vi "DataTransmissionActions.vi"(0 "Action":T2(ring), 1 "Transmission State In":T3(ring), 5 "Port Number In":dbl, 7 "Channel Names In":string[](array[string]), 9 "Time String":string, 11 "error in (no error)":errorcluster, 12 "Total Data In":dbl[](array[numeric]), 13 "Contol\nPoint\nSuffix":T1) -> (3 "Transmission State Out":T3(ring), 4 "Enabled":bool, 6 "Port Number Out":dbl, 10 "Channel Names Out":string[](array[string]), 14 "Stepwise Flag":bool, 15 "error out":errorcluster)   [LabVIEW 2009]
uses:
  lib/NTCP Client/Control Point Suffix.ctl
  Xmt Data.ctl
  DataTransmissionGlobals.vi
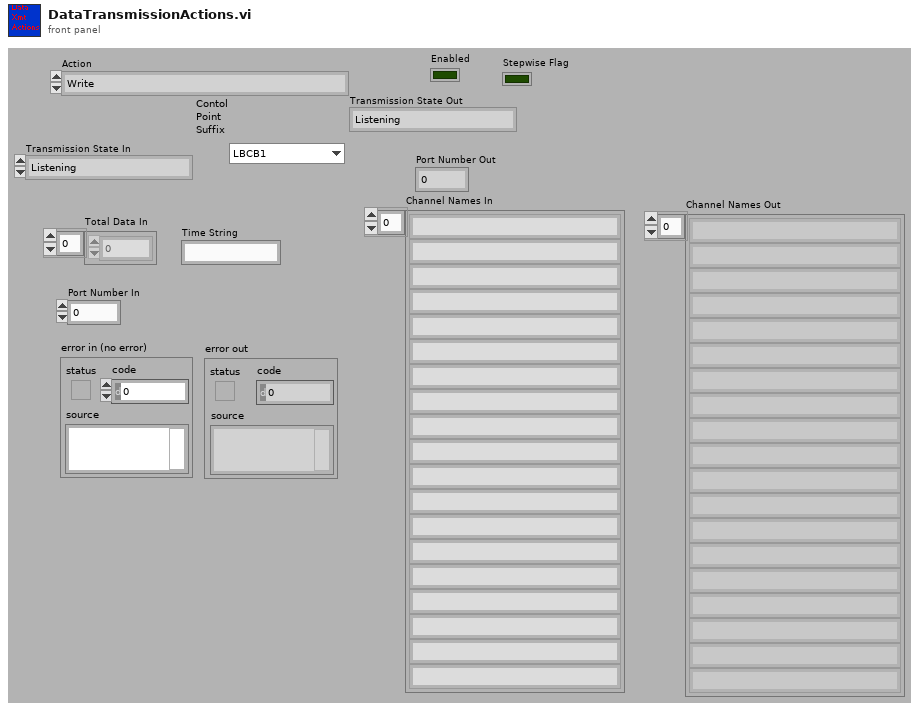
[diagram p1: front panel]
types:
  T1 = typedef "Control Point Suffix.ctl" = enum16{"LBCB1", "LBCB2", "ExternalSensors"}
  T2 = enum16{"Write", "Enable", "Disable", "Get Enabled", "Set Port Number", "Get Port Number", "Set Transmission State", "Get Tranmission State", "Set Channel Names", "Get Channel Names", "Set Stepwise Flag", "Clear Stepwise Flag", "Get Stepwise Flag"}
  T3 = enum16{"Listening", "Initializing", "Transmitting", "Disconnecting"}
  T4 = typedef "Xmt Data.ctl" = cluster{"Data":dbl[], "Time String":string, "Contol\nPoint\nSuffix":T1}
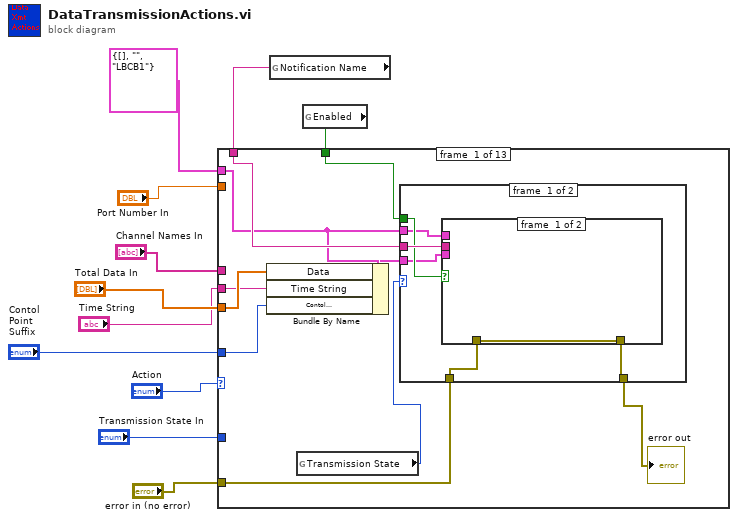
[diagram p0: block diagram]
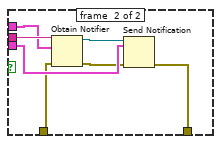
[diagram p2: hidden frame]
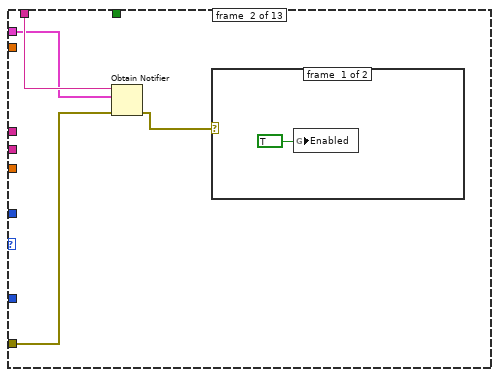
[diagram p4: hidden frame]
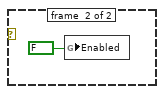
[diagram p5: hidden frame]
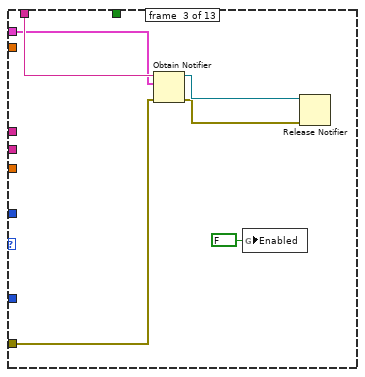
[diagram p6: hidden frame]
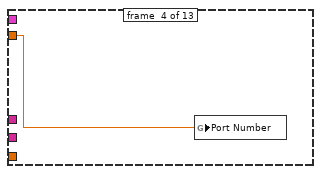
[diagram p7: hidden frame]
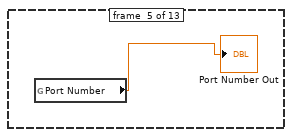
[diagram p8: hidden frame]
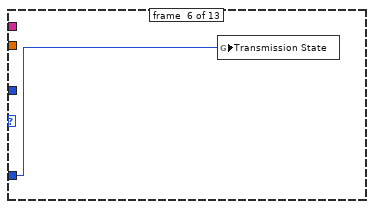
[diagram p9: hidden frame]
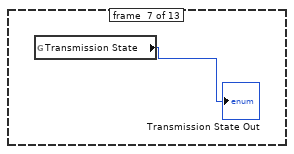
[diagram p10: hidden frame]
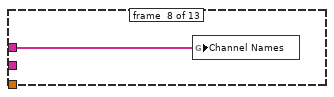
[diagram p11: hidden frame]
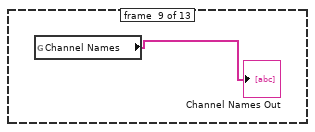
[diagram p12: hidden frame]
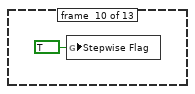
[diagram p13: hidden frame]
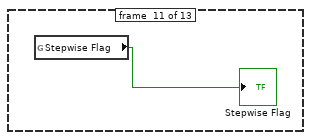
[diagram p14: hidden frame]
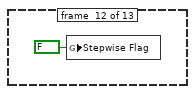
[diagram p15: hidden frame]
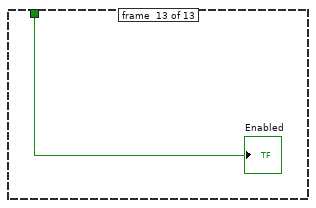
[diagram p16: hidden frame]
diagram:
  n1 = global read "DataTransmissionGlobals.vi" "Notification Name"() -> (w9:string)
  n2 = global read "DataTransmissionGlobals.vi" "Enabled"() -> (w5:bool)
  n3 = case shown="\"Write\", Default" "Action" {
    tunnel: "Total Data In" -> [w15 _ _ _ _ _ _ _ _ _ _ _ _]
    tunnel: w9 -> [w21 w40 w47 _ _ _ _ _ _ _ _ _ _]
    tunnel: "Port Number In" -> [_ _ _ w49 _ _ _ _ _ _ _ _ _]
    tunnel: "Transmission State In" -> [_ _ _ _ _ w51 _ _ _ _ _ _ _]
    tunnel: "error in (no error)" -> [w19 w39 w45 _ _ _ _ _ _ _ _ _ _]
    tunnel: w5 -> [w18 _ _ _ _ _ _ _ _ _ _ _ w58]
    tunnel: "Channel Names In" -> [_ _ _ _ _ _ _ w53 _ _ _ _ _]
    tunnel: T4 {"Data"=[], "Time String"="", "Contol\nPoint\nSuffix"=enum."LBCB1"} ("Xmt Data") -> [w16 w37 w43 _ _ _ _ _ _ _ _ _ _]
    tunnel: "Time String" -> [w14 _ _ _ _ _ _ _ _ _ _ _ _]
    tunnel: "Contol\nPoint\nSuffix" -> [w12 _ _ _ _ _ _ _ _ _ _ _ _]
    frame #0 {
      n4 = Bundle By Name(cluster=w16, "Data"=w15, "Time String"=w14, "Contol\nPoint\nSuffix"=w12) -> (w13:T4)
      n5 = global read "DataTransmissionGlobals.vi" "Transmission State"() -> (w20:T3)
      n6 = case shown="\"Transmitting\"" w20 {
        tunnel: w21 -> [w27 _]
        tunnel: w19 -> [w26 w36]
        tunnel: [w25 w36] -> w17
        tunnel: w18 -> [w24 _]
        tunnel: w16 -> [w23 _]
        tunnel: w13 -> [w22 _]
        frame #0 {
          n7 = case shown="True" w24 {
            tunnel: w27 -> [_ w34]
            tunnel: w22 -> [_ w33]
            tunnel: w26 -> [w28 w32]
            tunnel: [w28 w30] -> w25
            tunnel: w23 -> [_ w29]
            frame #0 {
            }
            frame #1 {
              n8 = Obtain Notifier(name (unnamed)=w34, notification data type=w29, error in (no error)=w32) -> (notifier out=w35:refnum<notifier>, error out=w31:errorcluster)  [unwired: 1 in, 1 out]
              n9 = Send Notification(notification=w33, notifier=w35, error in (no error)=w31) -> (error out=w30:errorcluster)  [unwired: 1 out]
            }
          }
        }
        frame #1 {
        }
      }
      "error out" <- w17
    }
    frame #1 {
      n10 = Obtain Notifier(name (unnamed)=w40, notification data type=w37, error in (no error)=w39) -> (error out=w38:errorcluster)  [unwired: 1 in, 2 out]
      n11 = case shown="No Error" w38 {
        frame #0 {
          n12 = global write "DataTransmissionGlobals.vi" "Enabled"(TRUE) -> ()
        }
        frame #1 {
          n13 = global write "DataTransmissionGlobals.vi" "Enabled"(FALSE) -> ()
        }
      }
    }
    frame #2 {
      n14 = Obtain Notifier(name (unnamed)=w47, notification data type=w43, error in (no error)=w45) -> (notifier out=w46:refnum<notifier>, error out=w44:errorcluster)  [unwired: 1 in, 1 out]
      n15 = global write "DataTransmissionGlobals.vi" "Enabled"(FALSE) -> ()
      n16 = Release Notifier(notifier=w46, error in (no error)=w44) -> ()  [unwired: 4 out]
    }
    frame #3 {
      n17 = global write "DataTransmissionGlobals.vi" "Port Number"(w49) -> ()
    }
    frame #4 {
      n18 = global read "DataTransmissionGlobals.vi" "Port Number"() -> (→"Port Number Out":dbl)
    }
    frame #5 {
      n19 = global write "DataTransmissionGlobals.vi" "Transmission State"(w51) -> ()
    }
    frame #6 {
      n20 = global read "DataTransmissionGlobals.vi" "Transmission State"() -> (→"Transmission State Out":T3)
    }
    frame #7 {
      n21 = global write "DataTransmissionGlobals.vi" "Channel Names"(w53) -> ()
    }
    frame #8 {
      n22 = global read "DataTransmissionGlobals.vi" "Channel Names"() -> (→"Channel Names Out":string[])
    }
    frame #9 {
      n23 = global write "DataTransmissionGlobals.vi" "Stepwise Flag"(TRUE ("Stepwise Flag")) -> ()
    }
    frame #10 {
      n24 = global read "DataTransmissionGlobals.vi" "Stepwise Flag"() -> (→"Stepwise Flag":bool)
    }
    frame #11 {
      n25 = global write "DataTransmissionGlobals.vi" "Stepwise Flag"(FALSE ("Stepwise Flag")) -> ()
    }
    frame #12 {
      "Enabled" <- w58
    }
  }
